vi "Verify Trim toque 45.vi"(6 "error in":errorcluster, 8 "MaxRead":i32, 9 "Channel in":u16) -> (0 "error out":errorcluster, 1 "Messages":T1(array[cluster]), 2 "Pass":bool, 3 "Channel out":u16)   [LabVIEW 2023]
uses:
  daf79331-edb1-4423-8e39-327e2c4704bb.vi
  57138545-9434-49a5-ae43-5830d40555d7.vi
  c1a646ff-5691-45d7-9623-f12d10756ac6.vi
  Communication/PCAN2023/PCAN API.lvlib
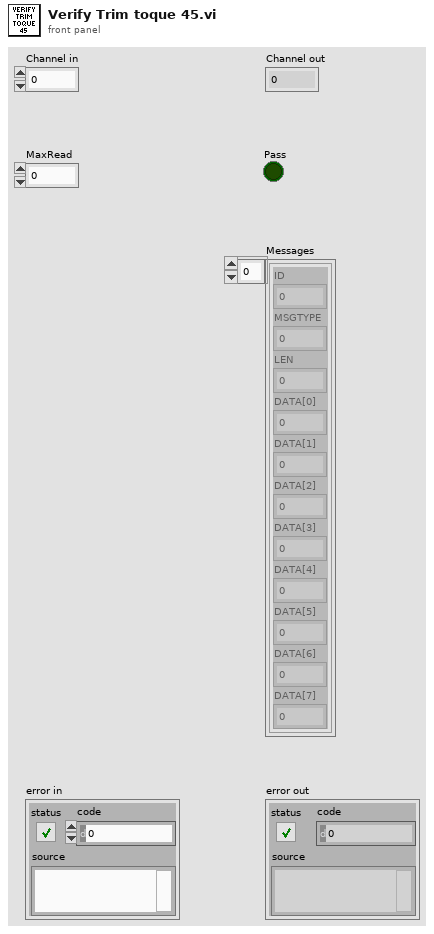
[diagram p1: front panel]
types:
  T1 = cluster{"ID":u32, "MSGTYPE":u8, "LEN":u8, "DATA[0]":u8, "DATA[1]":u8, "DATA[2]":u8, "DATA[3]":u8, "DATA[4]":u8, "DATA[5]":u8, "DATA[6]":u8, "DATA[7]":u8}[]
  T2 = cluster{"ID":u32, "MSGTYPE":u8, "LEN":u8, "DATA[0]":u8, "DATA[1]":u8, "DATA[2]":u8, "DATA[3]":u8, "DATA[4]":u8, "DATA[5]":u8, "DATA[6]":u8, "DATA[7]":u8}
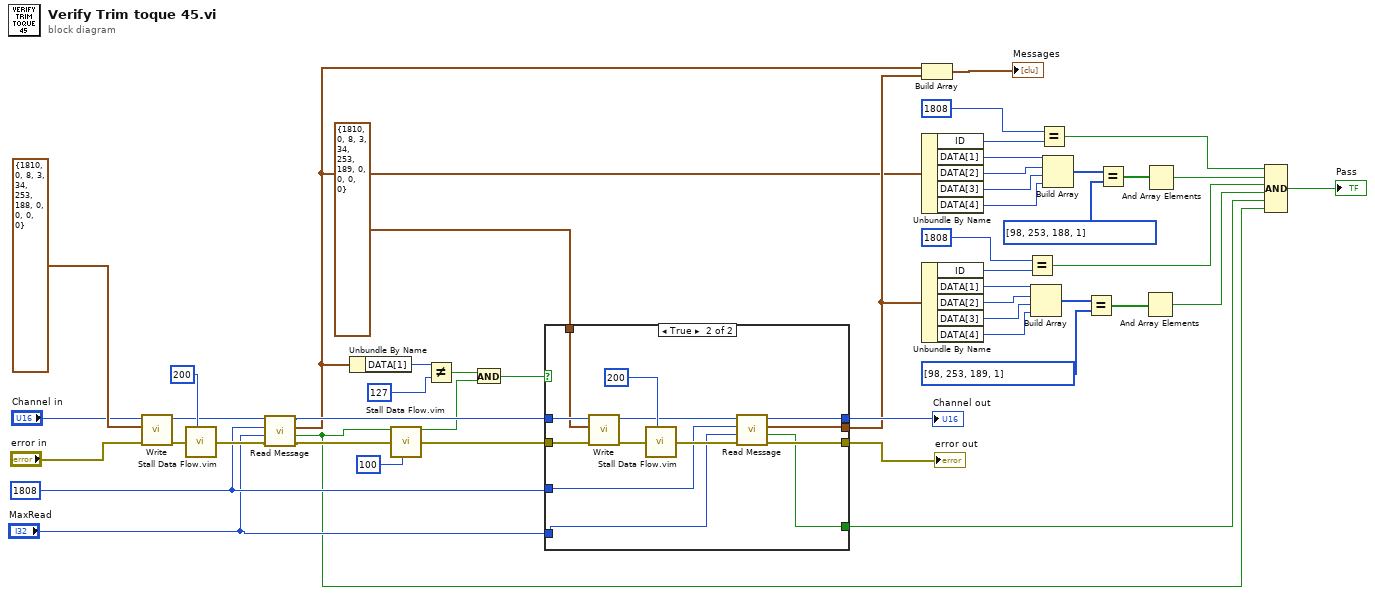
[diagram p0: block diagram]
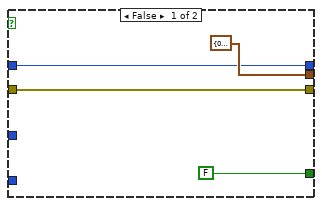
[diagram p2: hidden frame]
diagram:
  w8 = u32 1808 ("ID")
  n1 = call "Write.vi"("error in"="error in", "MessageBuffer"=T2 {"ID"=1810, "MSGTYPE"=0, "LEN"=8, "DATA[0]"=3, "DATA[1]"=34, "DATA[2]"=253, "DATA[3]"=188, "DATA[4]"=0, "DATA[5]"=0, "DATA[6]"=0, "DATA[7]"=0}, "Channel"="Channel in") -> ("error out"=w47:errorcluster, "Channel out"=w11:u16)  [unwired: 5 in, 2 out]
  n2 = call "Stall Data Flow.vim"("value in"=w47, "milliseconds to wait"=u32 200) -> ("value out"=w10:errorcluster)  [unwired: 1 out]
  n3 = call "Read Message.vi"("error in"=w10, "MaxRead"="MaxRead", "ID"=w8, "Channel in"=w11) -> ("error out"=w9:errorcluster, "Passed"=w2:bool, "Last Message"=w6:T2, "Channel out"=w7:u16)  [unwired: 3 in, 1 out]
  n4 = Unbundle By Name(w6) -> ("DATA[1]"=w12:u8)
  n5 = call "Stall Data Flow.vim"("value in"=w9, "milliseconds to wait"=u32 100) -> ("value out"=w41:errorcluster)  [unwired: 1 out]
  n6 = Not Equal?(x=w12, y=u8 127) -> (x != y?=w3:bool)
  n7 = And(x=w3, y=w2) -> (x .and. y?=w1:bool)
  n8 = case shown="True" w1 {
    tunnel: w7 -> [w51 w64]
    tunnel: [w51 w59] -> w44
    tunnel: [w50 w58] -> w43
    tunnel: T2 {"ID"=1810, "MSGTYPE"=0, "LEN"=8, "DATA[0]"=3, "DATA[1]"=34, "DATA[2]"=253, "DATA[3]"=189, "DATA[4]"=0, "DATA[5]"=0, "DATA[6]"=0, "DATA[7]"=0} ("MessageBuffer") -> [_ w63]
    tunnel: w8 -> [_ w56]
    tunnel: w41 -> [w50 w62]
    tunnel: [T2 {"ID"=0, "MSGTYPE"=0, "LEN"=0, "DATA[0]"=0, "DATA[1]"=0, "DATA[2]"=0, "DATA[3]"=0, "DATA[4]"=0, "DATA[5]"=0, "DATA[6]"=0, "DATA[7]"=0} ("MessageBuffer out") w54] -> w15
    tunnel: "MaxRead" -> [_ w55]
    tunnel: [FALSE ("Passed") w53] -> w4
    frame False {
    }
    frame True {
      n9 = call "Write.vi"("error in"=w62, "MessageBuffer"=w63, "Channel"=w64) -> ("error out"=w65:errorcluster, "Channel out"=w60:u16)  [unwired: 5 in, 2 out]
      n10 = call "Stall Data Flow.vim"("value in"=w65, "milliseconds to wait"=u32 200) -> ("value out"=w57:errorcluster)  [unwired: 1 out]
      n11 = call "Read Message.vi"("error in"=w57, "MaxRead"=w55, "ID"=w56, "Channel in"=w60) -> ("error out"=w58:errorcluster, "Passed"=w53:bool, "Last Message"=w54:T2, "Channel out"=w59:u16)  [unwired: 3 in, 1 out]
    }
  }
  "error out" <- w43
  "Channel out" <- w44
  n12 = Build Array(w6, w15) -> (→"Messages":T1)
  n13 = Unbundle By Name(w6) -> ("ID"=w34:u32, "DATA[1]"=w38:u8, "DATA[2]"=w37:u8, "DATA[3]"=w36:u8, "DATA[4]"=w35:u8)
  n14 = Unbundle By Name(w15) -> ("ID"=w27:u32, "DATA[1]"=w23:u8, "DATA[2]"=w24:u8, "DATA[3]"=w25:u8, "DATA[4]"=w26:u8)
  n15 = Equal?(x=u32 1808, y=w27) -> (x = y?=w22:bool)
  n16 = Build Array(w23, w24, w25, w26) -> (w29:u8[])
  n17 = Equal?(x=u32 1808, y=w34) -> (x = y?=w30:bool)
  n18 = Build Array(w38, w37, w36, w35) -> (w32:u8[])
  n19 = Equal?(x=w29, y=u8[] [98, 253, 189, 1]) -> (x = y?=w20:bool[])
  n20 = Equal?(x=w32, y=u8[] [98, 253, 188, 1]) -> (x = y?=w21:bool[])
  n21 = And Array Elements(Boolean array=w20) -> (logical AND=w18:bool)
  n22 = And Array Elements(Boolean array=w21) -> (logical AND=w19:bool)
  n23 = Compound Arithmetic op=AND(w30, w19, w22, w18, w4, w2) -> (→"Pass":bool)
